vi "PruebaTemp.vi"() -> ()   [LabVIEW 2014, in "MSX-E3711_dll.lvlib"]
uses:
  MSX-E3711_dll.lvlib
  Typedef/Connection Data.ctl
  Typedef/Config Data.ctl
  E:/Repositorio Magnis/INF002/v0/Modules/HAL/Drivers/Sync/ADDI-DATA MSX-E3711/API/MXCommon.dll
  MXCommon.dll
  E:/Repositorio Magnis/INF002/v0/Modules/HAL/Drivers/Sync/ADDI-DATA MSX-E3711/API/MSXE371x.dll
  MSXE371x.dll
panel:
  out "Temp Value":sgl
  in  "IncTemperature":T1
  out "error out":errorcluster
  in  "error in (no error)":errorcluster
  in  "Gain":bool
  in  "stop":bool
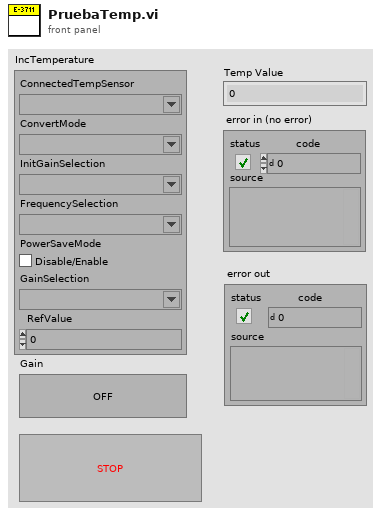
[diagram p1: front panel]
types:
  T1 = cluster{"ConnectedTempSensor":string, "ConvertMode":string, "InitGainSelection":string, "FrequencySelection":string, "PowerSaveMode":bool, "GainSelection":string, "RefValue":dbl}
  T2 = typedef "MSX-E3711_dll.lvlib/Config Data.ctl" = cluster{"Auto Refresh":cluster{"Average Mode":u64, "Average Value":u64, "Trigger Mask":u64, "Trigger Mode":u64, "Hardware Trigger Edge":u64, "Hardware Trigger Count":u64, "By Trigger Nbr Of Seq To Acquire":u64, "Time stamp":bool, "Analog Output(mm)":bool, "Invert value":bool, "Temperature value":bool, "Incremental counter value":bool, "Diff. mode":bool}, "Gain":sgl[], "Offset":sgl[], "Index":u64, "Range":sgl, "Sequence":cluster{"Nbr Of Sequence":u64, "Nbr Max Sequence To Transfer":u64, "Delay Mode":u64, "Delay Time Unit":u64, "Delay Value":u64, "Trigger Mask":u64, "Trigger Mode":u64, "Hardware Trigger Edge":u64, "Hardware Trigger Count":u64, "By Trigger Nbr Of Seq To Acquire":u64, "Time stamp":bool, "Sequence counter information":bool, "Analog Output(mm)":bool, "Invert value":bool, "Temperature value":bool, "Incremental counter value":bool, "Diff. mode":bool}, "Enable DIO":bool, "IncCounter":cluster{"CounterMode":string, "CounterOptionDIRECT  ":bool, "CounterOptionOthers":bool, "CounterClear ":bool}, "IncTemperature":cluster{"ConnectedTempSensor":string, "ConvertMode":string, "InitGainSelection":string, "FrequencySelection":string, "PowerSaveMode":bool, "GainSelection":string, "RefValue":dbl}}
  T3 = typedef "MSX-E3711_dll.lvlib/Connection Data.ctl" = cluster{"MX371x refnum":refnum<k24>, "IP":string, "Connection ID ":refnum<k5>, "MXCommon refnum":refnum<k24>}
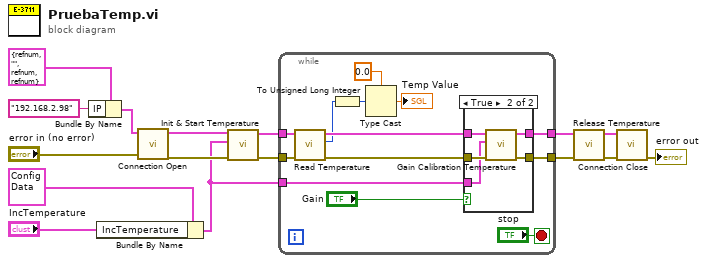
[diagram p0: block diagram]
diagram:
  n1 = Bundle By Name(cluster=T3 {"MX371x refnum"=refnum, "IP"="", "Connection ID "=refnum, "MXCommon refnum"=refnum} ("Connection Data In"), "IP"="192.168.2.98") -> (w5:T3)
  n2 = Bundle By Name(cluster=T2 {"Auto Refresh"={"Average Mode"=0, "Average Value"=0, "Trigger Mask"=0, "Trigger Mode"=0, "Hardware Trigger Edge"=0, "Hardware Trigger Count"=0, "By Trigger Nbr Of Seq To Acquire"=0, "Time stamp"=FALSE, "Analog Output(mm)"=FALSE, "Invert value"=FALSE, "Temperature value"=FALSE, "Incremental counter value"=FALSE, "Diff. mode"=FALSE}, "Gain"=[], "Offset"=[], "Index"=0, "Range"=0.0, "Sequence"={"Nbr Of Sequence"=0, "Nbr Max Sequence To Transfer"=800, "Delay Mode"=0, "Delay Time Unit"=0, "Delay Value"=0, "Trigger Mask"=5, "Trigger Mode"=0, "Hardware Trigger Edge"=0, "Hardware Trigger Count"=0, "By Trigger Nbr Of Seq To Acquire"=1, "Time stamp"=FALSE, "Sequence counter information"=TRUE, "Analog Output(mm)"=FALSE, "Invert value"=FALSE, "Temperature value"=FALSE, "Incremental counter value"=FALSE, "Diff. mode"=FALSE}, "Enable DIO"=FALSE, "IncCounter"={"CounterMode"="", "CounterOptionDIRECT  "=FALSE, "CounterOptionOthers"=FALSE, "CounterClear "=FALSE}, "IncTemperature"={"ConnectedTempSensor"="", "ConvertMode"="", "InitGainSelection"="", "FrequencySelection"="", "PowerSaveMode"=FALSE, "GainSelection"="", "RefValue"=0.0}} ("Config Data"), "IncTemperature"="IncTemperature") -> (w1:T2)
  n3 = call "Connection Open.vi"("error in (no error)"="error in (no error)", "Connection Data In"=w5) -> ("error out"=w15:errorcluster, "Connection Data Out"=w16:T3)  [unwired: 8 in]
  n4 = call "Init & Start Temperature.vi"("error in (no error)"=w15, "Config Data"=w1, "Connection Data In"=w16) -> ("error out"=w11:errorcluster, "Connection Data Out"=w12:T3)  [unwired: 7 in]
  n5 = while {
    tunnel: w12 -> [w28]
    tunnel: w11 -> [w27]
    tunnel: [w25] -> w10
    tunnel: [w23] -> w9
    tunnel: w1 -> [w21]
    stop <- "stop" stop-if-true
    n6 = call "Read Temperature.vi"("error in (no error)"=w27, "Connection Data In"=w28) -> ("error out"=w24:errorcluster, "TemperatureValue"=w20:u64, "Connection Data Out"=w26:T3)  [unwired: 7 in]
    n7 = To Unsigned Long Integer(number=w20) -> (unsigned 32bit integer=w19:u32)
    n8 = Type Cast(type=sgl 0.0, x=w19) -> (*(type *) &x=→"Temp Value":sgl)
    n9 = case shown="True" "Gain" {
      tunnel: w26 -> [w31 w36]
      tunnel: [w31 w35] -> w25
      tunnel: w24 -> [w30 w34]
      tunnel: [w30 w33] -> w23
      tunnel: w21 -> [_ w32]
      frame False {
      }
      frame True {
        n10 = call "Gain Calibration Temperature.vi"("error in (no error)"=w34, "Config Data"=w32, "Connection Data In"=w36) -> ("error out"=w33:errorcluster, "Connection Data Out"=w35:T3)  [unwired: 7 in]
      }
    }
  }
  n11 = call "Release Temperature.vi"("error in (no error)"=w9, "Connection Data In"=w10) -> ("error out"=w13:errorcluster, "Connection Data Out"=w14:T3)  [unwired: 8 in]
  n12 = call "Connection Close.vi"("error in (no error)"=w13, "Connection Data In"=w14) -> ("error out"=→"error out":errorcluster)  [unwired: 8 in, 1 out]
